vi "Requests.vi"(8 "error in (no error)":errorcluster, 9 "write enable":bool=TRUE, 11 "TEST in":refnum<class "TEST1.lvclass">) -> (0 "error out":errorcluster, 3 "TEST out":refnum<class "TEST1.lvclass">)   [LabVIEW 2021, in "TEST1.lvclass"]
uses:
  TEST1.lvclass
  D:/my_projects/projects/Algorithms/Labview/21/Modbus_v121c/Network Protocol/MB/Modbus Master CR.lvclass
  D:/my_projects/projects/Algorithms/Labview/21/Modbus_v121c/Network Protocol/Network Master/Network Master.lvclass
  MB/Modbus Master CR.lvclass/Modbus Master CR.ctl
  Modbus Data Unit/Modbus Data Unit.lvclass/Modbus Data Unit.ctl
  Network Protocol.lvclass/Network Protocol.ctl
  Network Master/Network Master.lvclass/Network Master.ctl
  Master Function Definition/Read Discrete Inputs Request.vi
  Network Master/Read write Master.vi
  Master Function Definition/Read Discrete Inputs Response.vi
  Master Function Definition/Read Input Registers Request.vi
  Master Function Definition/Read Input Registers Response.vi
  Master Function Definition/Write Multiple Coils Request.vi
  Master Function Definition/Function data mismatch error.vi
  Master Function Definition/Write Multiple Coils Response.vi
  Master Function Definition/Write Multiple Registers Request.vi
  Master Function Definition/Write Multiple Registers Response.vi
  Modbus Data Unit/Construct PDU.vi
  Read Transmission Data Unit.vi
  Utility/Bytes to Bits.vi
  Master Function Definition/Function code mismatch error.vi
  Data Model/Error Generator.vi
  Modbus Data Unit/Deconstruct PDU.vi
  Utility/Bytes to U16s.vi
  Utility/Bits to Bytes.vi
  Utility/U16s to Bytes.vi
  Network Master/Network Master.lvclass
  D:/my_projects/projects/Algorithms/Labview/21/Modbus_v121c/Network Protocol/Network Protocol.lvclass
  Modbus Data Unit/Modbus Data Unit.lvclass
  Data Model/Device Data Model.lvclass
  Transmission Data Unit/Transmission Data Unit.lvclass
  MB/Modbus Master CR.lvclass
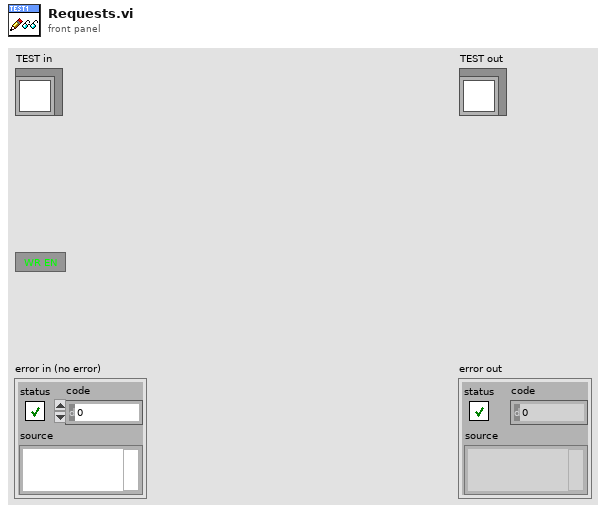
[diagram p1: front panel]
types:
  T1 = typedef "Modbus Master CR.lvclass/N channel.ctl" = cluster{"N DI channel":u16, "N DO channel":u16, "N AI channel":u16, "N AO channel":u16}
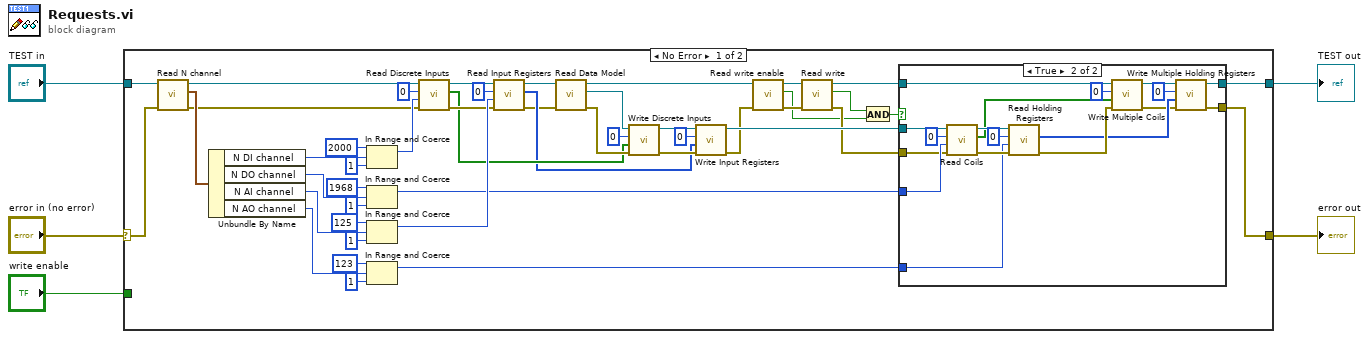
[diagram p0: block diagram]
diagram:
  n1 = case shown="No Error" "error in (no error)" {
    selector: "error in (no error)" -> [w49 w74]
    tunnel: [w16 w74] -> w3
    tunnel: [w15 w73] -> w4
    tunnel: "TEST in" -> [w50 w73]
    tunnel: "write enable" -> [_ _]
    frame No Error {
      n2 = call "Read N channel.vi"("error in (no error)"=w49, "MB_v2 in"=w50) -> ("error out"=w38:errorcluster, "N channel"=w51:T1, "MB_v2 out"=w44:refnum<class "TEST1.lvclass">)  [unwired: 7 in]
      n3 = Unbundle By Name(w51) -> ("N DI channel"=w43:u16, "N DO channel"=w29:u16, "N AI channel"=w35:u16, "N AO channel"=w32:u16)
      n4 = In Range and Coerce(upper limit=u16 2000, x=w43, lower limit=u16 1) -> (coerced(x)=w39:u16)  [unwired: 1 out]
      n5 = In Range and Coerce(upper limit=u16 1968, x=w29, lower limit=u16 1) -> (coerced(x)=w18:u16)  [unwired: 1 out]
      n6 = In Range and Coerce(upper limit=u16 125, x=w35, lower limit=u16 1) -> (coerced(x)=w28:u16)  [unwired: 1 out]
      n7 = In Range and Coerce(upper limit=u16 123, x=w32, lower limit=u16 1) -> (coerced(x)=w17:u16)  [unwired: 1 out]
      n8 = call "Read Discrete Inputs.vi"("error in (no error)"=w38, "number of discrete inputs"=w39, "starting address"=u16 0, "Modbus master in"=w44) -> ("error out"=w27:errorcluster, "discrete input values"=w25:bool[], "Modbus master out"=w26:refnum<class "TEST1.lvclass">)  [unwired: 5 in]
      n9 = call "Read Input Registers.vi"("error in (no error)"=w27, "number of input registers"=w28, "starting address"=u16 0, "Modbus master in"=w26) -> ("error out"=w21:errorcluster, "register values"=w22:u16[], "Modbus master out"=w20:refnum<class "TEST1.lvclass">)  [unwired: 5 in]
      n10 = call "Read Data Model.vi"("error in (no error)"=w21, "MB_TCP in"=w20) -> ("error out"=w47:errorcluster, "Data Model"=w46:refnum<class "Device Data Model.lvclass">, "MB_TCP out"=w12:refnum<class "TEST1.lvclass">)  [unwired: 7 in]
      n11 = call-dynamic "Write Discrete Inputs.vi"("error in (no error)"=w47, "input values"=w25, "starting address"=u16 0, "Device Data Model in"=w46) -> ("error out"=w23:errorcluster, "Device Data Model out"=w24:refnum<class "Device Data Model.lvclass">)  [unwired: 6 in]
      n12 = call-dynamic "Write Input Registers.vi"("error in (no error)"=w23, "register values"=w22, "starting address"=u16 0, "Device Data Model in"=w24) -> ("error out"=w13:errorcluster, "Device Data Model out"=w19:refnum<class "Device Data Model.lvclass">)  [unwired: 6 in]
      n13 = call "Read write enable.vi"("error in (no error)"=w13, "MB in"=w12) -> ("error out"=w10:errorcluster, "write enable"=w6:bool, "MB out"=w11:refnum<class "TEST1.lvclass">)  [unwired: 7 in]
      n14 = call "Read write.vi"("error in (no error)"=w10, "MB in"=w11) -> ("error out"=w9:errorcluster, "Write"=w8:bool, "MB out"=w7:refnum<class "TEST1.lvclass">)  [unwired: 7 in]
      n15 = And(x=w8, y=w6) -> (x .and. y?=w14:bool)
      n16 = case shown="True" w14 {
        tunnel: w19 -> [_ w72]
        tunnel: w18 -> [_ w67]
        tunnel: w17 -> [_ w66]
        tunnel: [w53 w58] -> w16
        tunnel: [w54 w57] -> w15
        tunnel: w9 -> [w53 w56]
        tunnel: w7 -> [w54 w55]
        frame False {
        }
        frame True {
          n17 = call-dynamic "Read Coils.vi"("error in"=w56, "number of coils"=w67, "starting address"=u16 0, "device data model in"=w72) -> ("error out"=w70:errorcluster, "data"=w64:bool[], "device data model out"=w71:refnum<class "Device Data Model.lvclass">)  [unwired: 5 in]
          n18 = call-dynamic "Read Holding Registers.vi"("error in"=w70, "number of registers"=w66, "starting address"=u16 0, "device data model in"=w71) -> ("error out"=w65:errorcluster, "data"=w60:u16[])  [unwired: 5 in, 1 out]
          n19 = call "Write Multiple Coils.vi"("error in (no error)"=w65, "coil values"=w64, "starting address"=u16 0, "Modbus master in"=w55) -> ("error out"=w59:errorcluster, "Modbus master out"=w62:refnum<class "TEST1.lvclass">)  [unwired: 6 in]
          n20 = call "Write Multiple Holding Registers.vi"("error in (no error)"=w59, "holding register values"=w60, "starting address"=u16 0, "Modbus master in"=w62) -> ("error out"=w58:errorcluster, "Modbus master out"=w57:refnum<class "TEST1.lvclass">)  [unwired: 6 in]
        }
      }
    }
    frame Error {
    }
  }
  "error out" <- w3
  "TEST out" <- w4
